vi "Play Stop Sound Effx.vi"(7 "Sound Effect":T1, 8 "Error In":errorcluster, 11 "Function":enum16{"Play", "Stop"}(ring)) -> (0 "error in (no error)":errorcluster)   [LabVIEW 2021, in "Sound Manager.lvlib"]
uses:
  Sound Manager.lvlib
  Typedefs/Sound Effects.ctl
  <vilib>/event_ctls.llb/usereventprio.ctl
  Architecture/Typedefs/Enum_Module_Name.ctl
  Architecture/Architecture.lvlib
  Architecture/Modules/Configuration/Configuration.lvlib
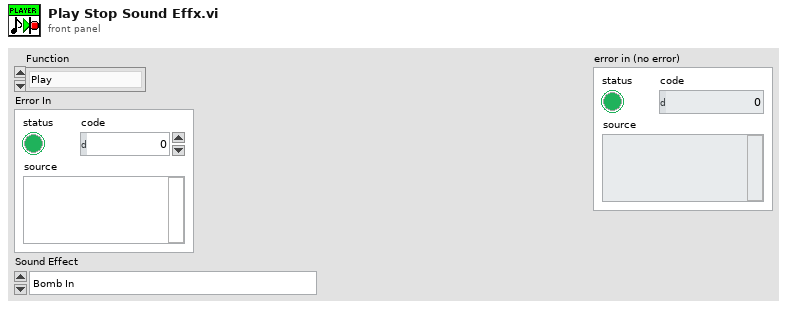
[diagram p1: front panel]
types:
  T1 = typedef "Sound Manager.lvlib/Sound Effects.ctl" = enum16{"Bomb In", "Bomb Out", "Bomb Touched", "Game Over", "Victory", "Eat", "10 Fruits", "Eat2", "Eat3", "Eat4", "MaxShield", "Shield", "10p", "Grape In", "Grape Out", "20p", "30p", "40p", "50p", "60p", "70p", "80p", "90p", "100p", "All shields cracked", "Mouse In", "Mouse Out", "Mouse Eaten", "Grape Eaten", "States Recover", "Broken Shield", "Bonus", "Happy Time", "explode", "Game over musica", "Back Music", "Shield Catch", "Evil lough", "Cricket In", "Cricket eaten", "Lets Go", "Jump1", "Jump2", "Jump3", "Unstoppable", "Troll Music", "winner", "menu"}
  T2 = typedef "Configuration.lvlib/Enum_Module_Name.ctl" = enum16{"Configuration", "Error_Handler", "Log", "Database", "Controller", "UI Module", "Sound Manager"}
  T3 = typedef "usereventprio.ctl" = enum32{"high priority", "normal priority"}
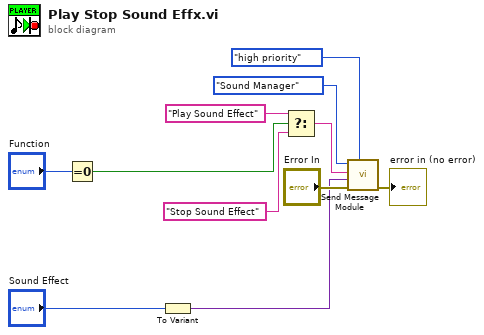
[diagram p0: block diagram]
diagram:
  n1 = Equal To 0?(x="Function") -> (x = 0?=w6:bool)
  n2 = To Variant(anything="Sound Effect") -> (Variant=w1:variant)
  n3 = Select(t="Play Sound Effect", s=w6, f="Stop Sound Effect") -> (s? t:f=w3:string)
  n4 = call "Send Message Module.vi"("priority (normal)"=usereventprio."high priority", "Error In"="Error In", "Data"=w1, "Message"=w3, "Target ModuleName In"=Enum_Module_Name."Sound Manager") -> ("error in (no error)"=→"error in (no error)":errorcluster)  [unwired: 6 in]
